vi "S2DS_Select User VI folder.vi"(11 "Path in":path) -> (1 "Folder selected?":bool, 3 "Path out":path)   [LabVIEW 2025]
panel:
  in  "Cancel":bool
  in  "OK":bool
  # "Please select your LabVIEW folder \n\ncontaining following files (exact match):\n     1. Users instruments inventory.vi\n     2. Users write instruments.vi\n     3. Users read instruments.vi"
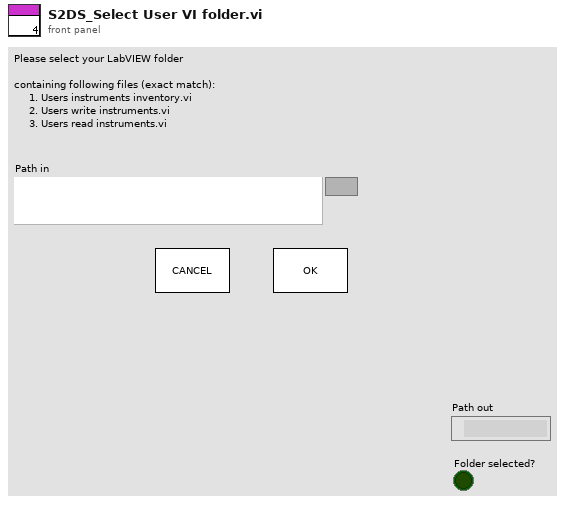
[diagram p1: front panel]
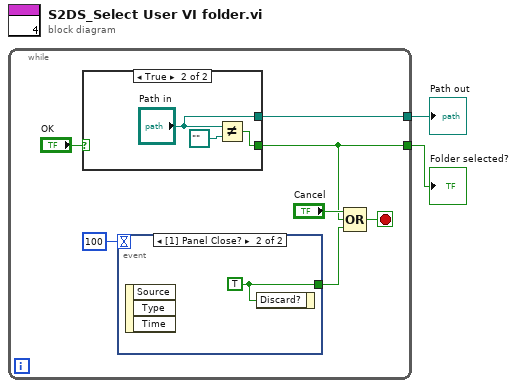
[diagram p0: block diagram]
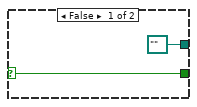
[diagram p2: hidden frame]
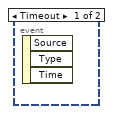
[diagram p3: hidden frame]
diagram:
  n1 = while {
    tunnel: [w5] -> w2
    tunnel: [w3] -> w1
    stop <- w9 stop-if-true
    n2 = case shown="True" "OK" {
      selector: "OK" -> [w10 _]
      tunnel: [path "" ("Path in") "Path in"] -> w5
      tunnel: [w10 w12] -> w3
      frame False {
      }
      frame True {
        n3 = Not Equal?(x="Path in", y=path "") -> (x != y?=w12:bool)
      }
    }
    n4 = event shown="[1] Panel Close?" {
      selector: _ -> [_ _]
      dyn-events: _ -> [_ _]
      timeout: 100 -> [_ _]
      tunnel: [_ w15] -> w7
      event Timeout {
        n5 = event-data() -> ()  [unwired: 1 in, 3 out]
      }
      event Panel Close? {
        w15 = TRUE ("Discard?")
        n6 = event-data() -> ()  [unwired: 1 in, 3 out]
        n7 = event-data("Discard?"=w15) -> ()  [unwired: 1 in, 1 out]
      }
    }
    n8 = Compound Arithmetic op=OR("Cancel", w3, w7) -> (w9:bool)
  }
  "Path out" <- w2
  "Folder selected?" <- w1
